vi "Suite from Project.vi"(8 "error in (no error)":errorcluster, 10 "Project Path":path, 11 "LUnit Test Suite In":refnum<class "LUnit Test Suite.lvclass">) -> (0 "error out":errorcluster, 3 "LUnit Test Suite Out":refnum<class "LUnit Test Suite.lvclass">)   [LabVIEW 2020, in "Test Finder.lvclass"]
doc: "Produce a test suite including all tests in a .lvproj file. This works recursively for nested projects."
uses:
  Test Finder.lvclass
  Test Finder.lvclass/Test Finder.ctl
  LUnit Test Suite.lvclass
  C:/git/astemes-lunit/source/Runnable.lvclass
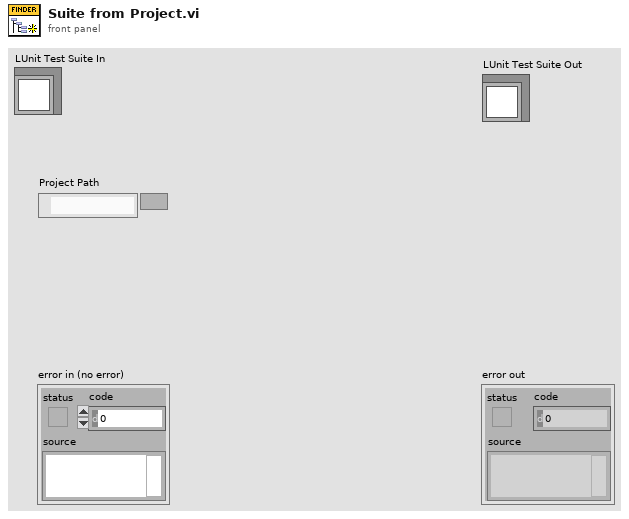
[diagram p1: front panel]
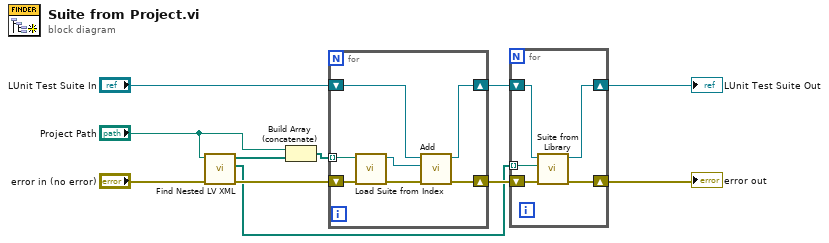
[diagram p0: block diagram]
diagram:
  n1 = call "Find Nested LV XML.vi"("error in (no error)"="error in (no error)", "Projext Path"="Project Path") -> ("error out"=w5:errorcluster, "lvlibs"=w1:path[], "lvprojs"=w7:path[])  [unwired: 7 in]
  n2 = Build Array (concatenate)("Project Path", w7) -> (w6:path[])
  n3 = for {
    tunnel: w6 -> [w14] mode=indexing
    shift-right: [w13] -> w3
    shift-left: "LUnit Test Suite In" -> [w17]
    shift-right: [w12] -> w9
    shift-left: w5 -> [w15]
    n4 = call "Load Suite from Index.vi"("error in (no error)"=w15, "Path"=w14) -> ("error out"=w16:errorcluster, "LUnit Test Suite out"=w18:refnum<class "LUnit Test Suite.lvclass">)  [unwired: 8 in]
    n5 = call "Add.vi"("error in (no error)"=w16, "Runnable"=w18, "LUnit Test Suite In"=w17) -> ("error out"=w12:errorcluster, "LUnit Test Suite Out"=w13:refnum<class "LUnit Test Suite.lvclass">)  [unwired: 7 in]
  }
  n6 = for {
    shift-right: [w22] -> w4
    shift-left: w9 -> [w23]
    shift-right: [w20] -> w2
    shift-left: w3 -> [w21]
    tunnel: w1 -> [w19] mode=indexing
    n7 = call "Suite from Library.vi"("error in (no error)"=w23, "Library Path"=w19, "LUnit Test Suite In"=w21) -> ("error out"=w22:errorcluster, "LUnit Test Suite Out"=w20:refnum<class "LUnit Test Suite.lvclass">)  [unwired: 7 in]
  }
  "error out" <- w4
  "LUnit Test Suite Out" <- w2
